vi "1.feladat.vi"() -> ()   [LabVIEW 2015]
panel:
  out "km/h":dbl
  in  "m/s":dbl
  out "Boolean 2":bool
  in  "Boolean":bool
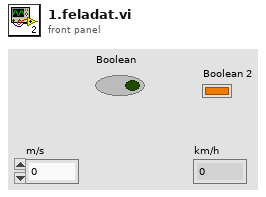
[diagram p1: front panel]
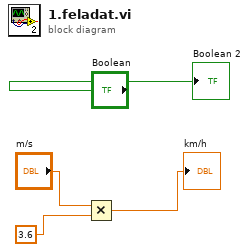
[diagram p0: block diagram]
diagram:
  n1 = Multiply(x="m/s", y=3.6) -> (x*y=→"km/h":dbl)
  "Boolean 2" <- "Boolean"
